vi "Read Digital Voltmeter.vi"(8 "error in (no error)":errorcluster, 11 "VISA resource name":refnum<visa-resource-name>) -> (0 "error out":errorcluster, 1 "Digital Voltmeter Frequency":dbl, 2 "Digital Voltmeter Value":dbl, 3 "VISA resource name out":refnum<visa-resource-name>)   [LabVIEW 2017, in "Scope.lvlib" / "Tektronix DPO MSO 2000 4000 Series.lvlib"]
doc: "Reads the current value and frequency for the Digital Voltmeter.\n\n<B>Notes:</B>\n(1) This VI is available for MDO3000 Series only.\n\n(2) Requires option MDO3DVM to be installed."
uses:
  Tektronix DPO MSO 2000 4000 Series.lvlib
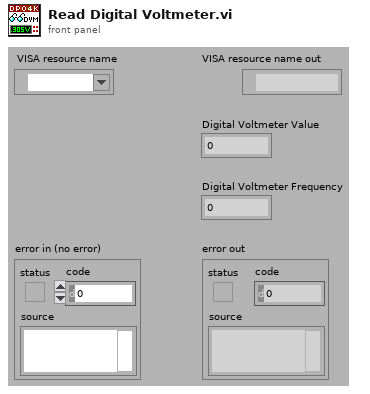
[diagram p1: front panel]
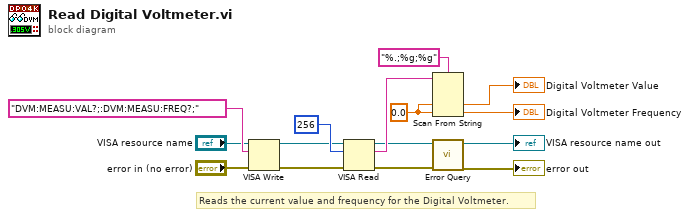
[diagram p0: block diagram]
diagram:
  w11 = 0.0 ("default value 1")
  # "Reads the current value and frequency for the Digital Voltmeter."
  n1 = VISA Write(VISA resource name="VISA resource name", write buffer="DVM:MEASU:VAL?;:DVM:MEASU:FREQ?;", error in (no error)="error in (no error)") -> (VISA resource name out=w2:refnum<visa-resource-name>, error out=w1:errorcluster)  [unwired: 1 out]
  n2 = VISA Read(VISA resource name=w2, byte count=u32 256, error in (no error)=w1) -> (VISA resource name out=w6:refnum<visa-resource-name>, read buffer=w10:string, error out=w5:errorcluster)  [unwired: 1 out]
  n3 = Scan From String(format string="%.;%g;%g", input string=w10, default 1=w11, default 2=w11) -> (output 1=→"Digital Voltmeter Value":dbl, output 2=→"Digital Voltmeter Frequency":dbl)  [unwired: 2 in, 3 out]
  n4 = call "Error Query.vi"("error in (no error)"=w5, "VISA resource name"=w6) -> ("error out"=→"error out":errorcluster, "VISA resource name out"=→"VISA resource name out":refnum<visa-resource-name>)  [unwired: 6 in, 2 out]
